vi "Acquire Data.vi"(8 "error in (no error)":errorcluster, 11 "Configuration Settings":T1={"Offset"=0.0, "Signal Type"=enum."Sine Wave", "Frequency"=10.0, "Amplitude"=1.0, "Phase"=0.0, "Noise Amplitude"=1.0} {"Noise Amplitude" format="%.2p"; "Phase" format="%.2p"; "Amplitude" format="%0.2p"; "Frequency" format="%0.2p"; "Offset" format="%0.2p"}) -> (0 "error out":errorcluster, 3 "Data Out":dbl[](array[numeric]))   [LabVIEW 2015]
uses:
  <vilib>/measure/NI_MABase.lvlib
  controls/Configuration Settings.ctl
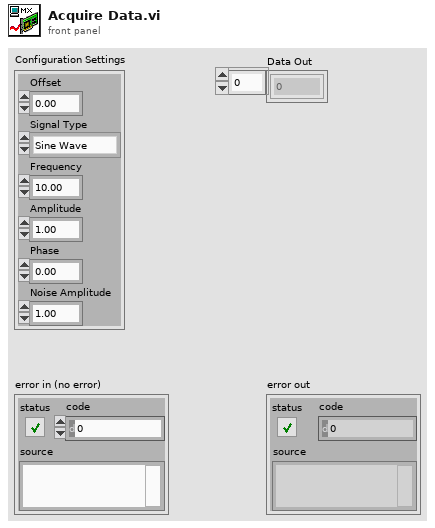
[diagram p1: front panel]
types:
  T1 = typedef "Configuration Settings.ctl" = cluster{"Offset":dbl, "Signal Type":enum16{"Sine Wave", "Triangle Wave", "Square Wave", "Sawtooth Wave"}, "Frequency":dbl, "Amplitude":dbl, "Phase":dbl, "Noise Amplitude":dbl}
  T2 = enum16{"Sine Wave", "Triangle Wave", "Square Wave", "Sawtooth Wave"}
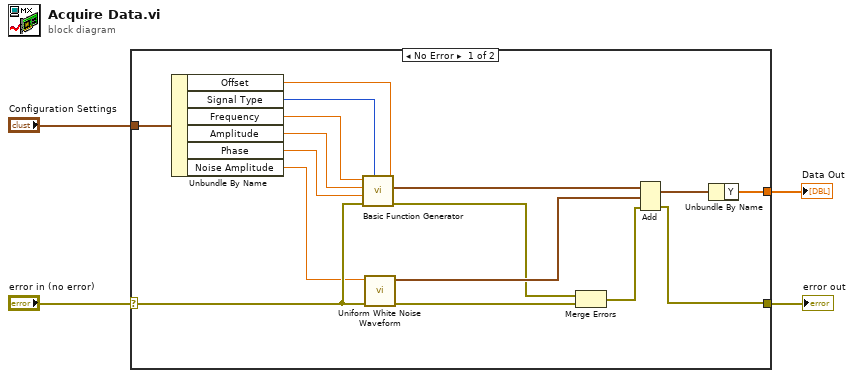
[diagram p0: block diagram]
diagram:
  n1 = case shown="No Error" "error in (no error)" {
    selector: "error in (no error)" -> [w15 w21]
    tunnel: [w18 w21] -> w3
    tunnel: [w16 _] -> w2
    tunnel: "Configuration Settings" -> [w11 _]
    frame No Error {
      n2 = Unbundle By Name(w11) -> ("Offset"=w5:dbl, "Signal Type"=w6:T2, "Frequency"=w7:dbl, "Amplitude"=w8:dbl, "Phase"=w9:dbl, "Noise Amplitude"=w10:dbl)
      n3 = call <vilib>:"Basic Function Generator.vi"("offset"=w5, "signal type"=w6, "error in (no error)"=w15, "phase"=w9, "amplitude"=w8, "frequency"=w7) -> ("error out"=w14:errorcluster, "signal out"=w20:waveform(dbl))  [unwired: 3 in, 1 out]
      n4 = call <vilib>:"Uniform White Noise Waveform.vi"("error in (no error)"=w15, "amplitude"=w10) -> ("error out"=w13:errorcluster, "signal out"=w19:waveform(dbl))  [unwired: 8 in]
      n5 = Merge Errors(w14, w13) -> (w12:errorcluster)
      n6 = Add(1:w19, 2:w20, 4:w12) -> (0:w17:waveform(dbl), 3:w18:errorcluster)
      n7 = Unbundle By Name(w17) -> ("Y"=w16:dbl[])
    }
    frame Error {
    }
  }
  "error out" <- w3
  "Data Out" <- w2
